vi "Speed_Set(SPD).vi"(5 "baud rate (9600)":u32=115200 caption="보 전송속도(9600)", 6 "Y SPEED":dbl format="%#_8g", 7 "X SPEED":dbl format="%#_8g", 8 "Port":refnum<visa-resource-name>="COM4" caption="VISA 리소스 이름") -> (2 "에러 출력":errorcluster, 3 "VISA 리소스 이름 출력":refnum<visa-resource-name>, 4 "연결된 문자열":string)   [LabVIEW 2010]
uses:
  <vilib>/Instr/_visa.llb/VISA Flush IO Buffer Mask.ctl
  <vilib>/Instr/_visa.llb/VISA Configure Serial Port (Instr).vi
panel:
  out "Read Buffer":string
  out "Write data":u32
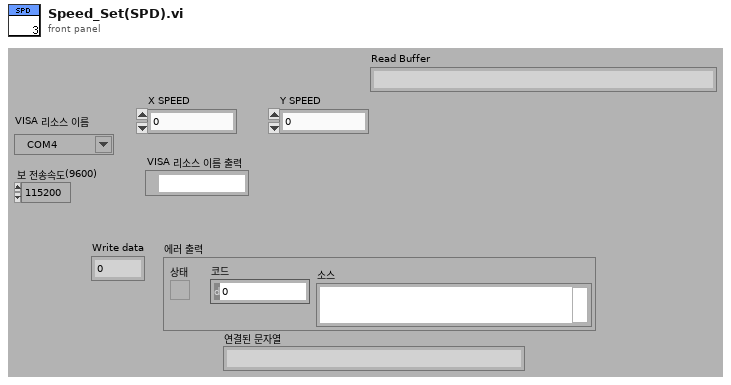
[diagram p1: front panel]
types:
  T1 = typedef "VISA Flush IO Buffer Mask.ctl" = u16
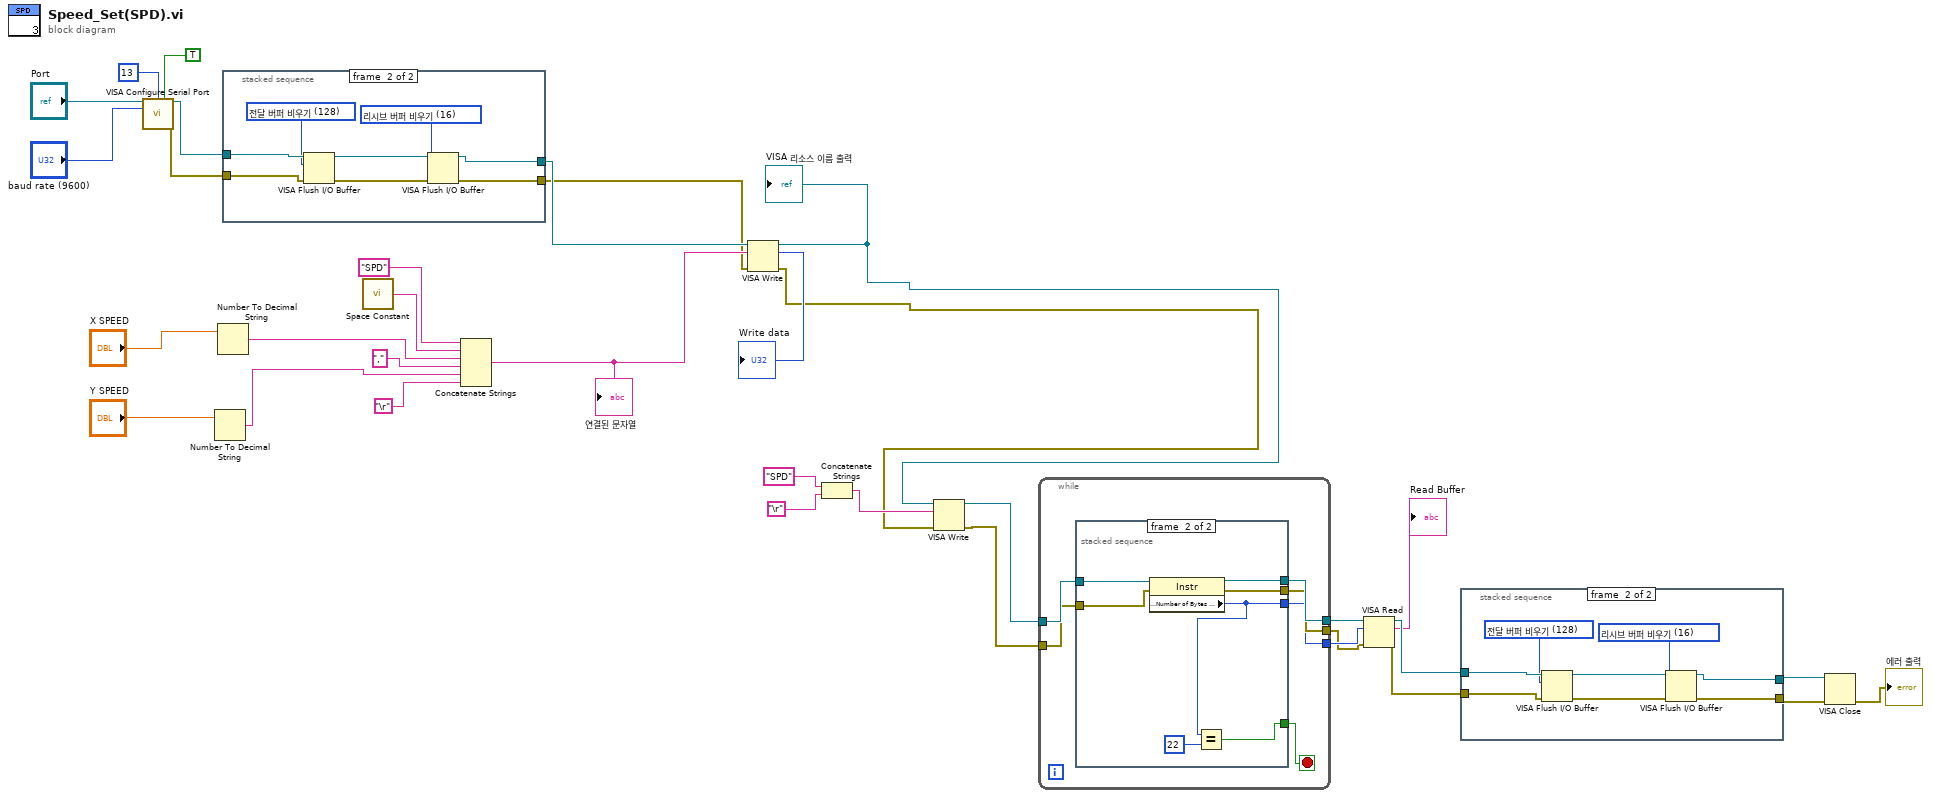
[diagram p0: block diagram]
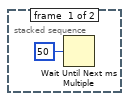
[diagram p2: hidden frame]
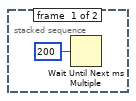
[diagram p3: hidden frame]
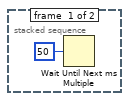
[diagram p4: hidden frame]
diagram:
  n1 = call-poly "VISA Configure Serial Port"("VISA resource name"="Port", "termination char\n(0xA = '\\n' = LF)"=i16 13 ("termination char\n(0xA = '\\n' = LF)"), "Enable Termination\nChar (T)"=TRUE ("Enable Termination\nChar (T)"), "baud rate (9600)"="baud rate (9600)") -> ("VISA resource name out"=w20:refnum<visa-resource-name>, "error out"=w19:errorcluster)  [unwired: 10 in]
  n2 = Number To Decimal String(number="Y SPEED") -> (decimal integer string=w26:string)  [unwired: 1 in]
  n3 = Number To Decimal String(number="X SPEED") -> (decimal integer string=w28:string)  [unwired: 1 in]
  n4 = stacked-sequence {
    tunnel: w20 -> [_ w43]
    tunnel: w19 -> [_ w42]
    tunnel: [_ w38] -> w18
    tunnel: [_ w37] -> w17
    frame #0 {
      n5 = Wait Until Next ms Multiple(millisecond multiple=u32 50 ("ms 배수")) -> ()  [unwired: 1 out]
    }
    frame #1 {
      w36 = T1 16 items=["리시브 버퍼 비우기"=16, "전달 버퍼 디바이스에 쓰기"=32, "리시브 버퍼 비우기(I/O 없음)"=64, "전달 버퍼 비우기"=128] ("Mask")
      w41 = T1 128 items=["리시브 버퍼 비우기"=16, "전달 버퍼 디바이스에 쓰기"=32, "리시브 버퍼 비우기(I/O 없음)"=64, "전달 버퍼 비우기"=128] ("Mask")
      n6 = VISA Flush I/O Buffer(VISA resource name=w43, mask (16)=w41, error in (no error)=w42) -> (VISA resource name out=w40:refnum<visa-resource-name>, error out=w39:errorcluster)
      n7 = VISA Flush I/O Buffer(VISA resource name=w40, mask (16)=w36, error in (no error)=w39) -> (VISA resource name out=w38:refnum<visa-resource-name>, error out=w37:errorcluster)
    }
  }
  n8 = call <vilib>:"Space Constant.vi"() -> ("String"=w29:string)
  n9 = Concatenate Strings("SPD" ("버퍼 쓰기"), w29, w28, "," ("문자열"), w26, "\r") -> (w32:string)
  "연결된 문자열" <- w32
  n10 = VISA Write(VISA resource name=w18, write buffer=w32, error in (no error)=w17) -> (VISA resource name out=w2:refnum<visa-resource-name>, return count=→"Write data":u32, error out=w1:errorcluster)
  "VISA 리소스 이름 출력" <- w2
  n11 = Concatenate Strings("SPD" ("버퍼 쓰기"), "\r") -> (w13:string)
  n12 = VISA Write(VISA resource name=w2, write buffer=w13, error in (no error)=w1) -> (VISA resource name out=w11:refnum<visa-resource-name>, error out=w10:errorcluster)  [unwired: 1 out]
  n13 = while {
    tunnel: w11 -> [w49]
    tunnel: w10 -> [w48]
    tunnel: [w47] -> w12
    tunnel: [w44] -> w5
    tunnel: [w46] -> w4
    stop <- w45 stop-if-true
    n14 = stacked-sequence {
      tunnel: w49 -> [_ w57]
      tunnel: w48 -> [_ w56]
      tunnel: [_ w55] -> w47
      tunnel: [_ w54] -> w46
      tunnel: [_ w52] -> w45
      tunnel: [_ w51] -> w44
      frame #0 {
        n15 = Wait Until Next ms Multiple(millisecond multiple=u32 200 ("ms 배수")) -> ()  [unwired: 1 out]
      }
      frame #1 {
        n16 = property class="Instr"(reference=w57, error in=w56) -> (reference out=w55:refnum<visa-resource-name>, error out=w54:errorcluster, "Serial Settings:Number of Bytes at Serial Port"=w51:u32)
        n17 = Equal?(x=w51, y=u32 22) -> (x = y?=w52:bool)
      }
    }
  }
  n18 = VISA Read(VISA resource name=w12, byte count=w5, error in (no error)=w4) -> (VISA resource name out=w9:refnum<visa-resource-name>, read buffer=→"Read Buffer":string, error out=w8:errorcluster)  [unwired: 1 out]
  n19 = stacked-sequence {
    tunnel: w9 -> [_ w66]
    tunnel: w8 -> [_ w65]
    tunnel: [_ w61] -> w7
    tunnel: [_ w60] -> w6
    frame #0 {
      n20 = Wait Until Next ms Multiple(millisecond multiple=u32 50 ("ms 배수")) -> ()  [unwired: 1 out]
    }
    frame #1 {
      w59 = T1 16 items=["리시브 버퍼 비우기"=16, "전달 버퍼 디바이스에 쓰기"=32, "리시브 버퍼 비우기(I/O 없음)"=64, "전달 버퍼 비우기"=128] ("Mask")
      w64 = T1 128 items=["리시브 버퍼 비우기"=16, "전달 버퍼 디바이스에 쓰기"=32, "리시브 버퍼 비우기(I/O 없음)"=64, "전달 버퍼 비우기"=128] ("Mask")
      n21 = VISA Flush I/O Buffer(VISA resource name=w66, mask (16)=w64, error in (no error)=w65) -> (VISA resource name out=w63:refnum<visa-resource-name>, error out=w62:errorcluster)
      n22 = VISA Flush I/O Buffer(VISA resource name=w63, mask (16)=w59, error in (no error)=w62) -> (VISA resource name out=w61:refnum<visa-resource-name>, error out=w60:errorcluster)
    }
  }
  n23 = VISA Close(VISA resource name=w7, error in (no error)=w6) -> (error out=→"에러 출력":errorcluster)
